vi "Begin Undo Transaction.vi"(7 "Transaction? (TRUE)":bool=TRUE, 8 "error in (no error)":errorcluster, 9 "Action":string, 11 "VI in":refnum<vi>) -> (0 "error out":errorcluster, 3 "VI out":refnum<vi>)   [LabVIEW 2020]
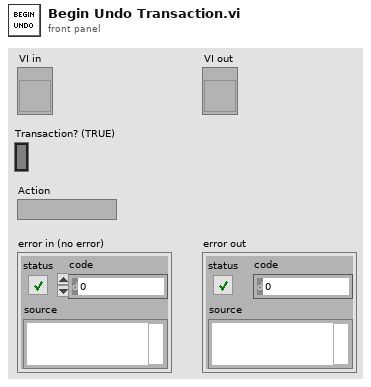
[diagram p1: front panel]
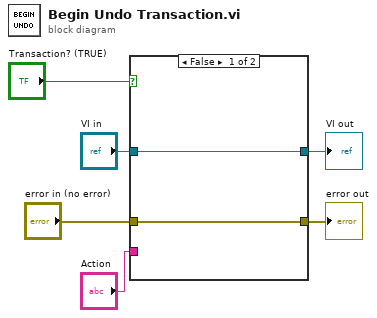
[diagram p0: block diagram]
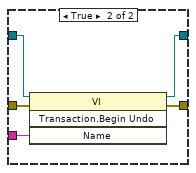
[diagram p2: hidden frame]
diagram:
  n1 = case shown="False" "Transaction? (TRUE)" {
    tunnel: "VI in" -> [w7 w13]
    tunnel: "error in (no error)" -> [w8 w12]
    tunnel: [w8 w11] -> w2
    tunnel: [w7 w10] -> w4
    tunnel: "Action" -> [_ w9]
    frame False {
    }
    frame True {
      n2 = invoke class="VI" method="Transaction.Begin Undo"(reference=w13, error in=w12, "Name"=w9) -> (reference out=w10:refnum<vi>, error out=w11:errorcluster)  [unwired: 1 in, 2 out]
    }
  }
  "VI out" <- w4
  "error out" <- w2
